vi "zoomedin3D.vi"() -> ()   [LabVIEW 2025]
uses:
  <vilib>/Analysis/1siggen.llb/Ramp Pattern by Samples.vi
  <vilib>/DAQmx/write.llb/DAQmx Write (Analog 1D Wfm NChan NSamp).vi
  <vilib>/DAQmx/read.llb/DAQmx Read (Counter 1D U32 1Chan NSamp).vi
  <vilib>/DAQmx/write.llb/DAQmx Write (Analog DBL 1Chan 1Samp).vi
  <vilib>/DAQmx/create/channels.llb/DAQmx Create Channel (AO-Voltage-Basic).vi
  <vilib>/DAQmx/configure/timing.llb/DAQmx Timing (Sample Clock).vi
  <vilib>/DAQmx/miscellaneous.llb/DAQmx Fill In Error Info.vi
  <vilib>/DAQmx/create/channels.llb/DAQmx Create Channel (CI-Count Edges).vi
  <vilib>/Analysis/NI_AALBase.lvlib
panel:
  in  "file (use dialog)":path
  out "Min Vy":dbl
  out "Max Vy":dbl
  out "Min Vx":dbl
  out "Max Vx":dbl
  out "Intensity Graph":dbl[][](graph)
  out "appended array":dbl[][](array[numeric])
  out "transposed array":dbl[][](array[numeric])
  out "64bit integer":i64[](array[numeric])
  in  "Dwell time (s)":dbl
  in  "new px":i32=128
  in  "Around desired spot":i32=128
  in  "Y coordinate":i32
  in  "X coordinate":i32
  in  "old px":i32=128
  in  "Volts":dbl=10.0 format="%0.2f"
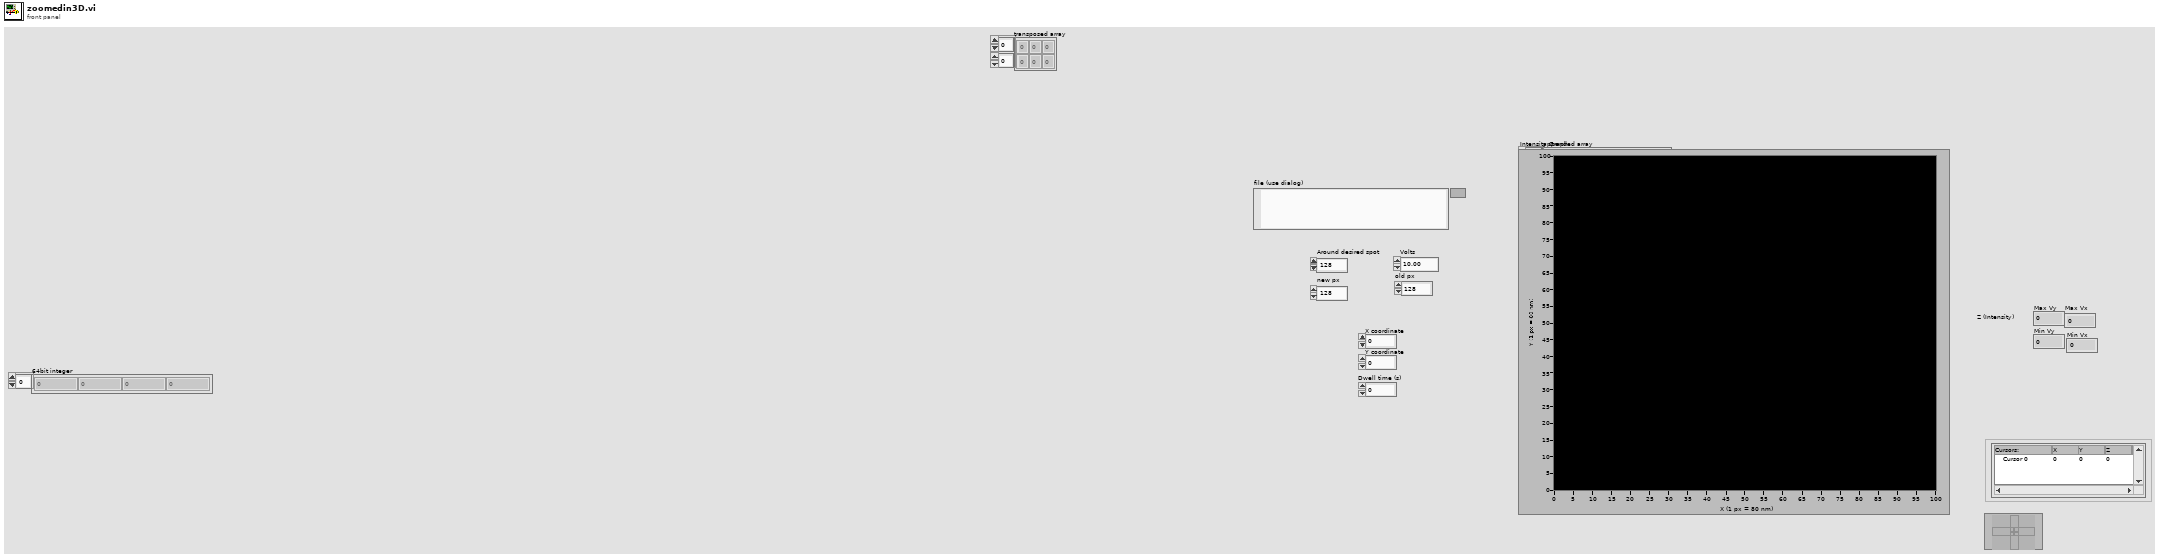
[diagram p1: front panel]
types:
  T1 = enum16{"big-endian, network order", "native, host order", "little-endian"}
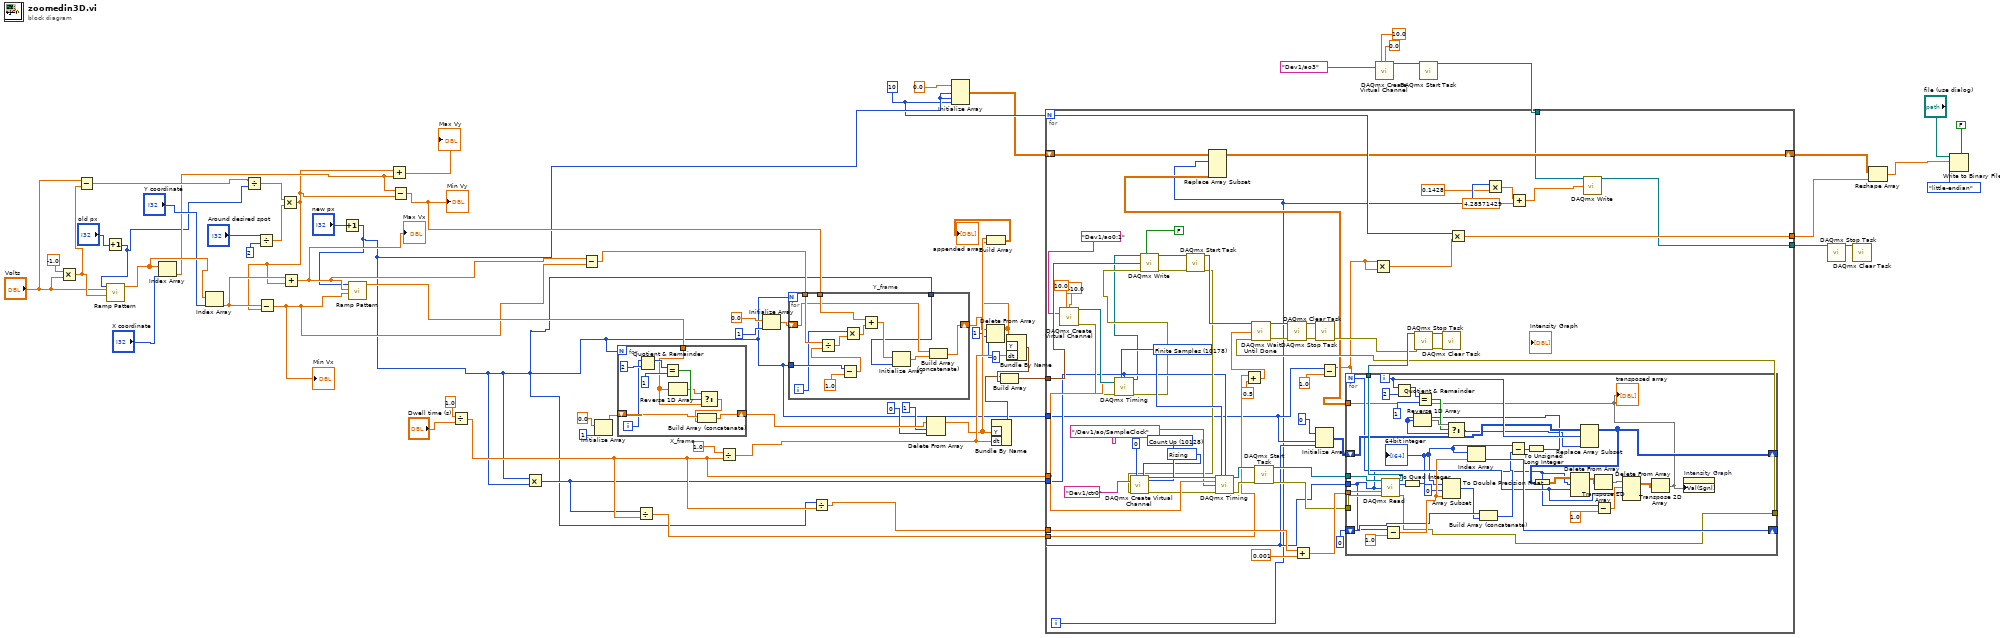
[diagram p0: block diagram]
diagram:
  w15 = 10 ("dimension size")
  n1 = Multiply(x=-1.0, y="Volts") -> (x*y=w60:dbl)
  n2 = Subtract(x="Volts", y=w60) -> (x-y=w58:dbl)
  n3 = Increment(x="old px") -> (x+1=w19:i32)
  n4 = call-poly <vilib>:"Ramp Pattern.vi"("start"=w60, "end"="Volts", "samples"=w19) -> ("Ramp Pattern"=w64:dbl[])  [unwired: 7 in, 1 out]
  n5 = Index Array(array=w64, index="X coordinate") -> (element=w24:dbl)
  n6 = Index Array(array=w64, index="Y coordinate") -> (element=w26:dbl)
  n7 = Divide(x=w58, y=w19) -> (x/y=w57:dbl)
  n8 = Divide(x="Around desired spot", y=2) -> (x/y=w56:dbl)
  n9 = Multiply(x=w57, y=w56) -> (x*y=w23:dbl)
  n10 = Subtract(x=w26, y=w23) -> (x-y=w21:dbl)
  "Min Vx" <- w21
  n11 = Add(x=w26, y=w23) -> (x+y=w25:dbl)
  "Max Vx" <- w25
  n12 = Increment(x="new px") -> (x+1=w16:i32)
  n13 = call-poly <vilib>:"Ramp Pattern.vi"("start"=w21, "end"=w25, "samples"=w16) -> ("Ramp Pattern"=w27:dbl[])  [unwired: 7 in, 1 out]
  n14 = Add(x=w23, y=w24) -> (x+y=→"Max Vy":dbl)
  n15 = Subtract(x=w24, y=w23) -> (x-y=w20:dbl)
  "Min Vy" <- w20
  n16 = Divide(x=1.0, y="Dwell time (s)") -> (x/y=w33:dbl)
  n17 = Multiply(x=w16, y=w16) -> (x*y=w31:i32)
  n18 = Subtract(x=w25, y=w21) -> (x-y=w29:dbl)
  n19 = Initialize Array(0.0 ("element"), 1 ("dimension size")) -> (w48:dbl[])
  n20 = for "X_frame" {
    N: w16 -> [_]
    shift-right: [w75] -> w41
    shift-left: w48 -> [w76]
    tunnel: w27 -> [w69]
    i -> [w70]
    n21 = Quotient & Remainder(x=w70, y=2) -> (x-y*floor(x/y)=w73:i32)  [unwired: 1 out]
    n22 = Equal?(x=w73, y=1) -> (x = y?=w71:bool)
    n23 = Reverse 1D Array(array=w69) -> (reversed array=w68:dbl[])
    n24 = Select(t=w68, s=w71, f=w69) -> (s? t:f=w67:dbl[])
    n25 = Build Array (concatenate)(w76, w67) -> (w75:dbl[])
  }
  n26 = Divide(x=w31, y=w33) -> (x/y=w30:dbl)
  n27 = Divide(x=1.0, y=w33) -> (x/y=w50:dbl)
  n28 = Initialize Array(0.0 ("element"), 1 ("dimension size")) -> (w49:dbl[])
  n29 = for "Y_frame" {
    N: w16 -> [_]
    tunnel: w16 -> [w89]
    tunnel: w29 -> [w87]
    tunnel: w20 -> [w82]
    tunnel: w16 -> [w77]
    shift-right: [w78] -> w37
    shift-left: w49 -> [w79]
    i -> [w84]
    n30 = Subtract(x=w89, y=1.0) -> (x-y=w86:dbl)
    n31 = Divide(x=w87, y=w86) -> (x/y=w85:dbl)
    n32 = Multiply(x=w84, y=w85) -> (x*y=w83:dbl)
    n33 = Add(x=w82, y=w83) -> (x+y=w81:dbl)
    n34 = Initialize Array(w81, w77) -> (w80:dbl[])
    n35 = Build Array (concatenate)(w79, w80) -> (w78:dbl[])
  }
  n36 = Divide(x=w16, y=w33) -> (x/y=w32:dbl)
  n37 = Delete From Array "Delete From Array"(array=w41, length=1, index=0) -> (array with subset deleted=w38:dbl[])  [unwired: 1 out]
  n38 = Initialize Array(0.0 ("element"), w16, w16, w15) -> (w14:dbl[][][])
  n39 = Delete From Array "Delete From Array"(array=w37, length=1, index=0) -> (array with subset deleted=w34:dbl[])  [unwired: 1 out]
  n40 = Build Array(w38, w34) -> (→"appended array":dbl[][])
  n41 = Bundle By Name("Y"=w38, "dt"=w50) -> (w51:waveform(dbl))  [unwired: 1 in]
  n42 = Bundle By Name("Y"=w34, "dt"=w50) -> (w52:waveform(dbl))  [unwired: 1 in]
  n43 = Build Array(w51, w52) -> (w53:waveform(dbl)[])
  n44 = call-poly <vilib>:"DAQmx Create Virtual Channel.vi"("maximum value"=10.0, "minimum value"=0.0, "physical channels"=tag "Dev1/ao3") -> ("task out"=w7:refnum<k21>)  [unwired: 11 in, 1 out]
  n45 = call <vilib>:"DAQmx Start Task.vi"("task/channels in"=w7) -> ("task out"=w4:refnum<k21>)  [unwired: 13 in, 1 out]
  n46 = for {
    N: w15 -> [w101]
    tunnel: w53 -> [w139]
    tunnel: w33 -> [w129]
    tunnel: w32 -> [w126]
    tunnel: w31 -> [w113]
    tunnel: w30 -> [w112]
    tunnel: w16 -> [w108]
    shift-right: [w100] -> w12
    shift-left: w14 -> [w103]
    tunnel: [w99] -> w11
    tunnel: w4 -> [w96]
    tunnel: [w95] -> w2
    i -> [w92]
    w145 = 10178 items=["Finite Samples"=10178, "Continuous Samples"=10123, "Hardware Timed Single Point"=12522] ("Sample mode")
    w135 = 10280 items=["Rising"=10280, "Falling"=10171] ("edge")
    w136 = 10128 items=["Count Up"=10128, "Count Down"=10124, "Externally Controlled"=10326] ("count direction")
    n47 = call-poly <vilib>:"DAQmx Create Virtual Channel.vi"("maximum value"=10.0, "minimum value"=-10.0, "physical channels"="Dev1/ao0:1" ("Galvo mirror path")) -> ("task out"=w138:refnum<k21>, "error out"=w124:errorcluster)  [unwired: 11 in]
    n48 = call-poly <vilib>:"DAQmx Timing.vi"("task/channels in"=w138, "sample mode"=w145, "samples per channel"=w113, "rate"=w129, "error in"=w124) -> ("task out"=w104:refnum<k21>, "error out"=w105:errorcluster)  [unwired: 9 in]
    n49 = call-poly <vilib>:"DAQmx Write.vi"("task/channels in"=w104, "auto start"=FALSE, "data"=w139, "error in"=w105) -> ("task out"=w140:refnum<k21>, "error out"=w123:errorcluster)  [unwired: 9 in, 1 out]
    n50 = call <vilib>:"DAQmx Start Task.vi"("task/channels in"=w140, "error in"=w123) -> ("task out"=w147:refnum<k21>, "error out"=w120:errorcluster)  [unwired: 12 in]
    n51 = call-poly <vilib>:"DAQmx Create Virtual Channel.vi"("initial count"=u32 0, "count direction"=w136, "edge"=w135, "counter"="Dev1/ctr0" ("Counter path"), "error in"=w120) -> ("task out"=w142:refnum<k21>, "error out"=w122:errorcluster)  [unwired: 9 in]
    n52 = call-poly <vilib>:"DAQmx Timing.vi"("task/channels in"=w142, "sample mode"=w145, "samples per channel"=w113, "rate"=w129, "source"=tag "/Dev1/ao/SampleClock", "error in"=w122) -> ("task out"=w143:refnum<k21>, "error out"=w121:errorcluster)  [unwired: 8 in]
    n53 = Add(x=w112, y=0.5) -> (x+y=w110:dbl)
    n54 = call <vilib>:"DAQmx Start Task.vi"("task/channels in"=w143, "error in"=w121) -> ("task out"=w144:refnum<k21>, "error out"=w115:errorcluster)  [unwired: 12 in]
    n55 = Add(x=w126, y=0.001) -> (x+y=w130:dbl)
    n56 = Initialize Array(u32 0 ("element"), w108, w108) -> (w146:u32[][])
    n57 = Subtract(x=w108, y=1.0) -> (x-y=w97:dbl)
    n58 = for {
      N: w97 -> [w157]
      tunnel: w108 -> [w154]
      tunnel: w130 -> [w184]
      tunnel: w144 -> [w183]
      shift-right: [w166] -> _
      shift-left: w146 -> [w169]
      tunnel: [w178] -> w125
      shift-right: [w175] -> _
      shift-left: u64 0 ("Numeric") -> [w173]
      tunnel: w115 -> [w164]
      tunnel: [w163] -> w114
      tunnel: [w151] -> w102
      i -> [w170]
      n59 = call-poly <vilib>:"DAQmx Read.vi"("task/channels in"=w183, "number of samples per channel"=w154, "timeout"=w184, "error in"=w164) -> ("task out"=w178:refnum<k21>, "data"=w165:u32[], "error out"=w163:errorcluster)  [unwired: 9 in]
      n60 = Subtract(x=w154, y=1.0) -> (x-y=w174:dbl)
      n61 = Quotient & Remainder(x=w170, y=2) -> (x-y*floor(x/y)=w181:i32)  [unwired: 1 out]
      n62 = To Quad Integer(1:w165) -> (0:w152:i64[])
      "64bit integer" <- w152
      n63 = Equal?(x=w181, y=1) -> (x = y?=w177:bool)
      n64 = Array Subset "Array Subset"(array=w152, index=0, length=w174) -> (w153:i64[])
      n65 = Index Array "Index Array"(array=w152, index=w174) -> (element=w175:i64)
      n66 = Build Array (concatenate) "Build Array"(w173, w153) -> (w172:u64[])
      n67 = Subtract(x=w152, y=w172) -> (x-y=w171:u64[])
      n68 = To Unsigned Long Integer(number=w171) -> (unsigned 32bit integer=w168:u32[])
      n69 = Reverse 1D Array(array=w168) -> (reversed array=w179:u32[])
      n70 = Select(t=w179, s=w177, f=w168) -> (s? t:f=w167:u32[])
      n71 = Replace Array Subset "Replace Array Subset"(array=w169, new element=w167, index (row)=w170) -> (w166:u32[][])  [unwired: 1 in]
      n72 = To Double Precision Float(number=w166) -> (double precision float=w162:dbl[][])
      n73 = Delete From Array(array=w162, length=w154, index (row)=w157) -> (array with subset deleted=w161:dbl[][])  [unwired: 1 in, 1 out]
      n74 = Transpose 2D Array(2D array=w161) -> (transposed array=w160:dbl[][])
      n75 = Subtract(x=w154, y=1.0) -> (x-y=w158:dbl)
      n76 = Delete From Array(array=w160, length=w158, index (row)=w157) -> (array with subset deleted=w156:dbl[][])  [unwired: 1 in, 1 out]
      n77 = Transpose 2D Array(2D array=w156) -> (transposed array=w151:dbl[][])
      "transposed array" <- w151
      n78 = property on="Intensity Graph" class="IntGraph (strict)"("Val(Sgnl)"=w151) -> ()  [unwired: 2 in, 2 out]
    }
    n79 = Replace Array Subset(array=w103, new element=w102, index (dim 0)=w92) -> (w100:dbl[][][])  [unwired: 2 in]
    n80 = call <vilib>:"DAQmx Wait Until Done.vi"("task/channels in"=w147, "timeout (sec)"=w110, "error in"=w114) -> ("task out"=w148:refnum<k21>, "error out"=w119:errorcluster)  [unwired: 11 in]
    n81 = call <vilib>:"DAQmx Stop Task.vi"("task/channels in"=w148, "error in"=w119) -> ("task out"=w141:refnum<k21>, "error out"=w118:errorcluster)  [unwired: 12 in]
    n82 = call <vilib>:"DAQmx Clear Task.vi"("task in"=w141, "error in"=w118) -> ("error out"=w117:errorcluster)  [unwired: 13 in]
    n83 = Multiply(x=w97, y=w97) -> (x*y=w98:dbl)
    n84 = call <vilib>:"DAQmx Stop Task.vi"("task/channels in"=w125, "error in"=w117) -> ("task out"=w149:refnum<k21>, "error out"=w116:errorcluster)  [unwired: 12 in]
    n85 = call <vilib>:"DAQmx Clear Task.vi"("task in"=w149, "error in"=w116) -> ()  [unwired: 13 in, 1 out]
    n86 = Multiply(x=w101, y=w98) -> (x*y=w99:dbl)
    n87 = Multiply(x=w92, y=0.1428) -> (x*y=w91:dbl)
    n88 = Add(x=w91, y=4.28571429) -> (x+y=w94:dbl)
    n89 = call-poly <vilib>:"DAQmx Write.vi"("task/channels in"=w96, "data"=w94) -> ("task out"=w95:refnum<k21>)  [unwired: 11 in, 2 out]
  }
  n90 = call <vilib>:"DAQmx Stop Task.vi"("task/channels in"=w2) -> ("task out"=w3:refnum<k21>)  [unwired: 13 in, 1 out]
  n91 = call <vilib>:"DAQmx Clear Task.vi"("task in"=w3) -> ()  [unwired: 14 in, 1 out]
  n92 = Reshape Array(w12, w11) -> (w10:dbl[])
  n93 = Write to Binary File(file (use dialog)="file (use dialog)", data=w10, 5:FALSE ("prepend array or string size? (T)"), 9:T1."little-endian" ("byte order (0:big-endian, network order)")) -> ()  [unwired: 2 in, 3 out]
